vi "AddReplaceChannel.vi"(8 "Channel In":T1[](array[typedef]), 11 "Channels in":T1[](array[typedef])) -> (3 "Channels out":T1[](array[typedef]))   [LabVIEW 2016, in "DCM-DSI.lvclass"]
uses:
  DCM-DSI.lvclass
  Channel.ctl
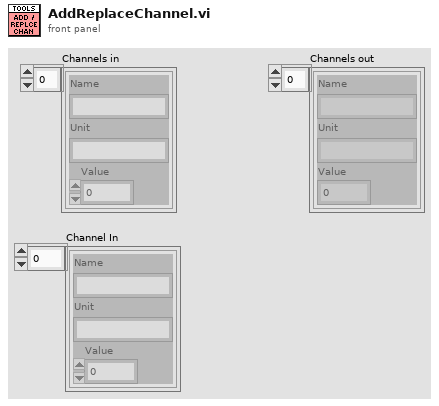
[diagram p1: front panel]
types:
  T1 = typedef "DCM-DSI.lvclass/Channel.ctl" = cluster{"Name":string, "Unit":string, "Value":sgl}
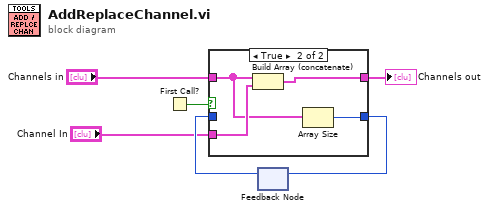
[diagram p0: block diagram]
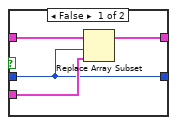
[diagram p2: hidden frame]
diagram:
  n1 = First Call?() -> (First Call?: T/F=w1:bool)
  n2 = feedback #1() -> (w6:i32)  [unwired: 1 in]
  n3 = case shown="True" w1 {
    tunnel: "Channels in" -> [w10 w11]
    tunnel: "Channel In" -> [w8 w14]
    tunnel: [w9 w13] -> w4
    tunnel: [w7 w12] -> w5
    tunnel: w6 -> [w7 _]
    frame False {
      n4 = Replace Array Subset(array=w10, new element=w8, index=w7) -> (w9:T1[])
    }
    frame True {
      n5 = Build Array (concatenate)(w11, w14) -> (w13:T1[])
      n6 = Array Size(array=w11) -> (size(s)=w12:i32)
    }
  }
  "Channels out" <- w4
  n7 = feedback-in #1(w5) -> ()
